vi "PARSER.vi"() -> ()   [LabVIEW 2010]
panel:
  out "HTTP Header":string
  out "Path":string
  out "Config":cluster{"OpenFP":bool, "UseAuthentication":bool}
  out "errors":errorcluster
  out "ControlIndicator":T1(array[cluster])
  out "vi reference":refnum<vi>
  out "SesionID":i32
  out "JIL-XMLversion":string="Version 0.1"
  out "STATE":T2(ring)
  out "Compatible utf8?":bool
  out "Commands recieved":i32
  out "IMPUT":string
  out "OUTPUT":string
  out "Error TCP":errorcluster
  in  "CloneRef":refnum<vi>
  in  "connection ID":refnum<k5>
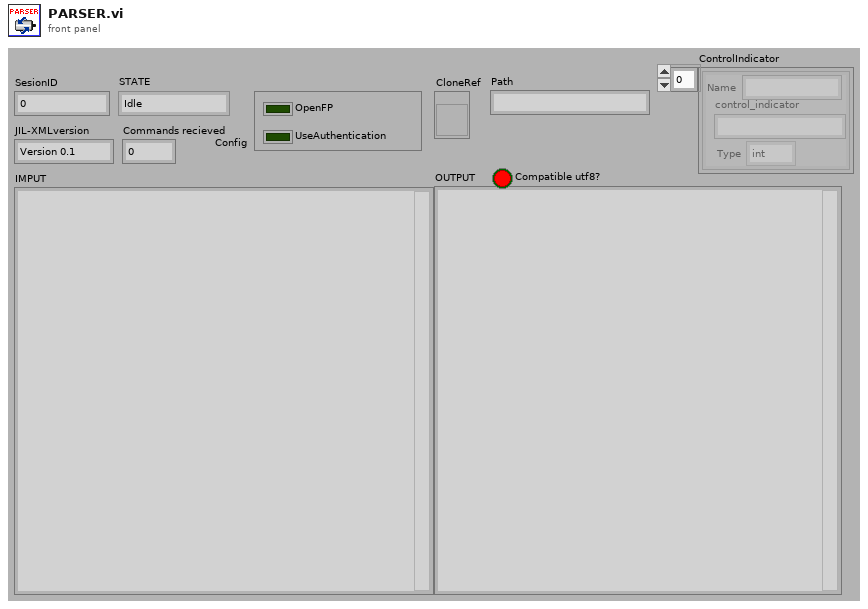
[diagram p1: front panel]
types:
  T1 = cluster{"Name":string, "control_indicator":string, "Type":enum16{"int", "boolean", "string", "double", "dateTime", "base64", "struct", "array"}}[]
  T2 = enum16{"Idle", "Connected", "Authenticated", "Opened", "Running", "Exit"}
  T3 = enum16{"Standard", "Buffered", "CRLF", "Immediate"}
  T4 = enum16{"Connect", "Authenticate", "OpenVI", "RunVI", "SyncVI", "StopVI", "CloseVI", "Disconnect"}
  T5 = enum16{"int", "boolean", "string", "double", "dateTime", "base64", "struct", "array"}
  T6 = enum16{"Update", "registry", "Init", "clean", "Close"}
  T7 = enum16{"int", "boolean", "string", "double", "dateTime", "base64", "struct", "array"}[]
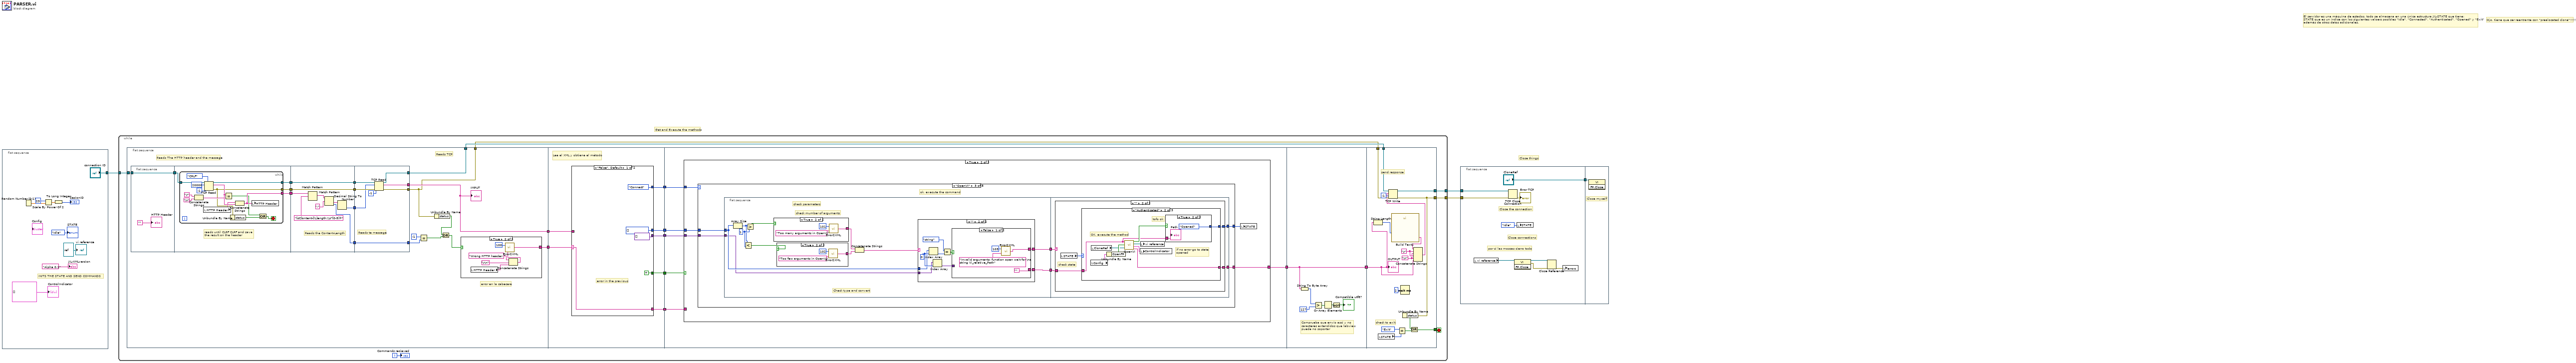
[diagram p0: block diagram]
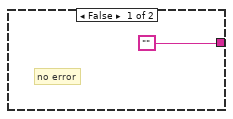
[diagram p2: hidden frame]
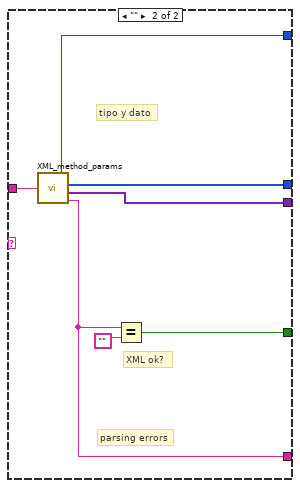
[diagram p3: hidden frame]
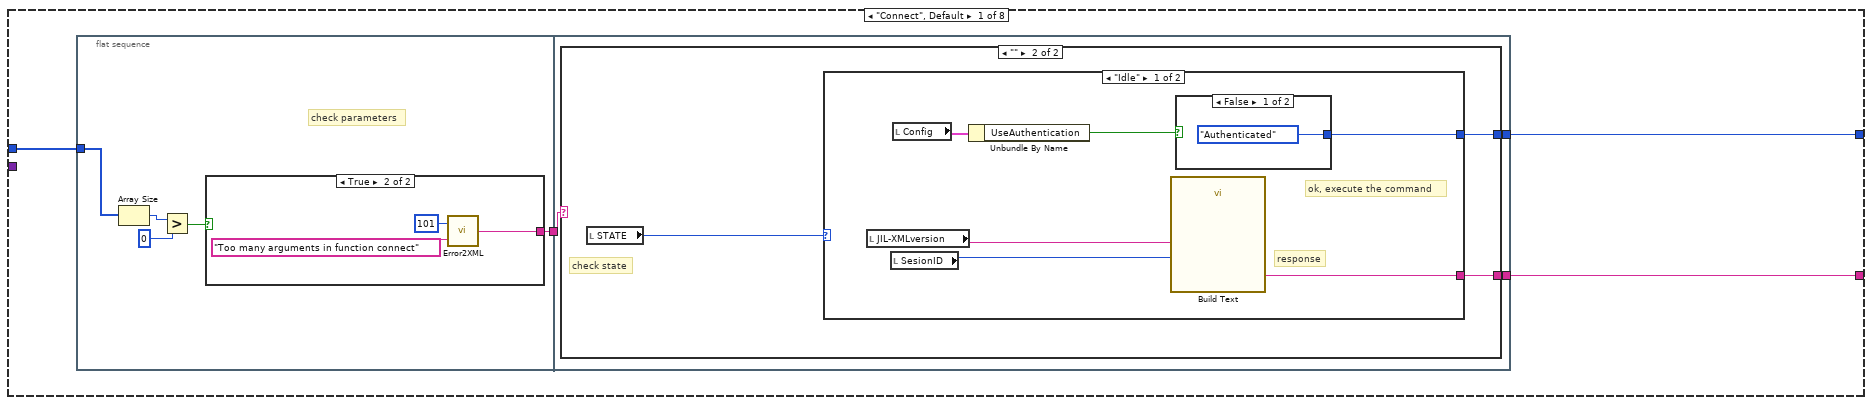
[diagram p5: hidden frame]
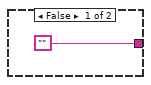
[diagram p6: hidden frame]
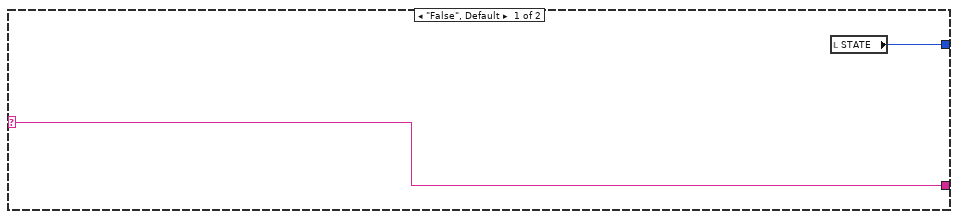
[diagram p7: hidden frame]
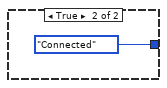
[diagram p8: hidden frame]
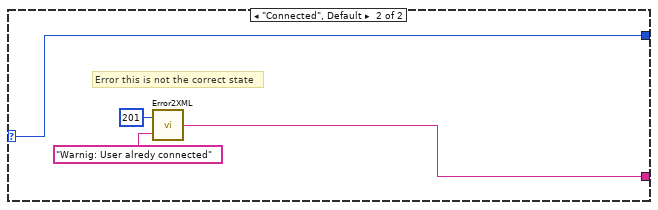
[diagram p9: hidden frame]
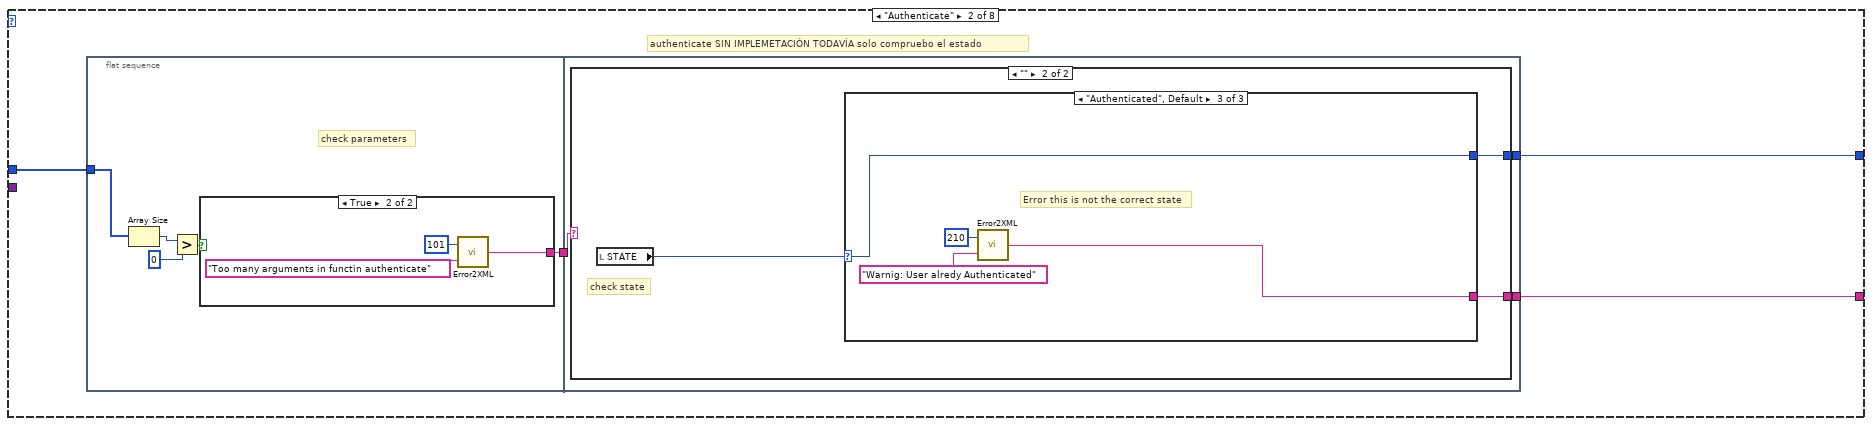
[diagram p10: hidden frame]
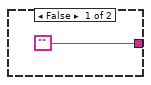
[diagram p11: hidden frame]
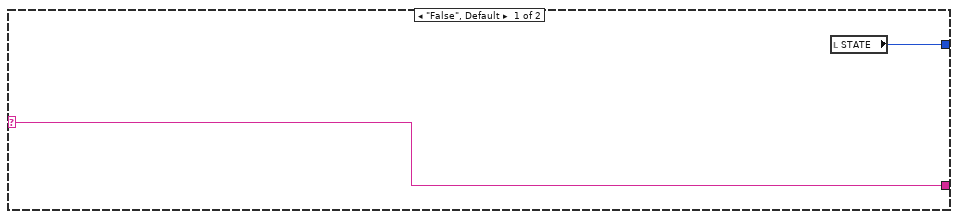
[diagram p12: hidden frame]
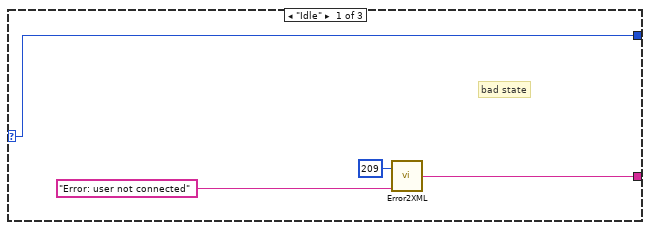
[diagram p13: hidden frame]
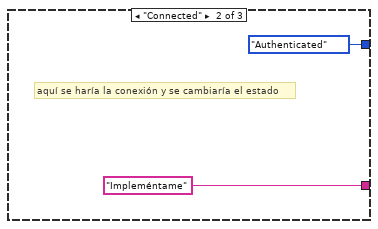
[diagram p14: hidden frame]
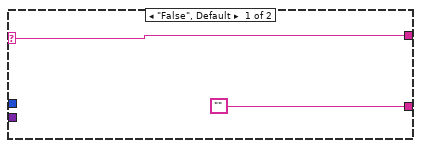
[diagram p15: hidden frame]
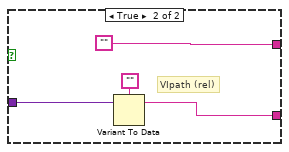
[diagram p16: hidden frame]
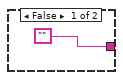
[diagram p17: hidden frame]
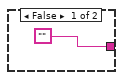
[diagram p18: hidden frame]
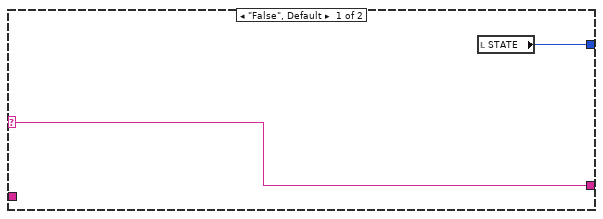
[diagram p19: hidden frame]
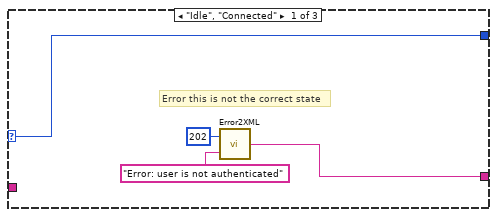
[diagram p20: hidden frame]
diagram:
  # "Close things"
  # "Get and Execute the methods"
  # "El servidor es una máquina de estados, todo se almacena en una única estructura JIL-STATE que tiene:\nSTATE que es un índice con los siguientes valoers posibles \"Idle\", \"Connected\", \"Authenticated\", \"Opened\" y \"Exit\"\nademás de otros datos adicionales."
  # "Ojo, tiene que ser reentrante con \"prealocated clone\"!!!!!!"
  n1 = flat-sequence {
    tunnel: ["connection ID"] -> w1
    frame #0 {
      # "INITS THE STATE AND SEND COMMANDS"
      n2 = Random Number (0-1)() -> (number: 0 to 1=w9:dbl)
      n3 = Scale By Power Of 2(n=23, x=w9) -> (x*2^n=w10:dbl)
      n4 = To Long Integer(number=w10) -> (32bit integer=→"SesionID":i32)
      "STATE" <- T2."Idle" ("STATE")
      "JIL-XMLversion" <- "Alpha 0.1" ("JIL-XMLversion")
      "vi reference" <- refnum<vi> refnum ("vi reference")
      "ControlIndicator" <- T1 [] ("ControlIndicator")
    }
  }
  n5 = while {
    tunnel: [w29] -> w3
    tunnel: [w26] -> w2
    tunnel: w1 -> [w15]
    i -> [w24]
    stop <- w27 stop-if-true
    n6 = flat-sequence {
      tunnel: [w39] -> w28
      tunnel: [w37] -> w25
      tunnel: [w38] -> w21
      tunnel: w15 -> [w47]
      tunnel: [w30] -> w14
      tunnel: [w95] -> w23
      tunnel: [w94] -> w22
      tunnel: w21 -> [w99]
      tunnel: [w98] -> w20
      tunnel: [w97] -> w18
      tunnel: [w96] -> w17
      tunnel: w14 -> [w93]
      tunnel: w23 -> [w117]
      tunnel: [w115] -> w19
      tunnel: w22 -> [w116]
      tunnel: w20 -> [w114]
      tunnel: w18 -> [w113]
      tunnel: w17 -> [w112]
      tunnel: w19 -> [w478]
      tunnel: [w478] -> w16
      tunnel: [w491] -> w29
      tunnel: w28 -> [w492]
      tunnel: [w495] -> w27
      tunnel: [w494] -> w26
      tunnel: w25 -> [w498]
      tunnel: w16 -> [w483]
      frame #0 {
        # "error en la cabecera"
        # "Reads The HTTP header and the message"
        # "Reads TCP"
        n7 = flat-sequence {
          tunnel: w47 -> [w55]
          tunnel: [w55] -> w46
          tunnel: w46 -> [w60]
          tunnel: [w59] -> w45
          tunnel: [w58] -> w42
          tunnel: [w57] -> w40
          tunnel: w45 -> [w84]
          tunnel: [w79] -> w44
          tunnel: [w78] -> w43
          tunnel: w42 -> [w78]
          tunnel: [w77] -> w41
          tunnel: w40 -> [w77]
          tunnel: [w76] -> w36
          tunnel: w44 -> [w89]
          tunnel: w43 -> [w90]
          tunnel: w41 -> [w91]
          tunnel: [w88] -> w39
          tunnel: [w87] -> w37
          tunnel: [w86] -> w38
          tunnel: [w85] -> w35
          tunnel: w36 -> [w85]
          frame #0 {
            "HTTP Header" <- ""
          }
          frame #1 {
            # "reads until CLRF CLRF and save \nthe result on the header"
            n8 = while {
              tunnel: w60 -> [w74]
              tunnel: [w66] -> w59
              tunnel: [w64] -> w58
              tunnel: [w65] -> w57
              stop <- w61 stop-if-true
              n9 = Concatenate Strings("\r", "\n") -> (w69:string)
              n10 = local read "HTTP Header"() -> (w70:string)
              n11 = TCP Read(connection ID=w74, bytes to read=20000, 7:T3."CRLF" ("mode (standard)"), 9:-1 ("timeout ms (25000)")) -> (connection ID out=w65:refnum<k5>, data out=w71:string, error out=w64:errorcluster)  [unwired: 1 in]
              n12 = Equal?(x=w71, y=w69) -> (x = y?=w63:bool)
              n13 = Unbundle By Name(w64) -> ("status"=w62:bool)
              n14 = Concatenate Strings(w70, w71) -> (w66:string)
              n15 = local write "HTTP Header"(w66) -> ()
              n16 = Or(x=w63, y=w62) -> (x .or. y?=w61:bool)
            }
          }
          frame #2 {
            # "Reads the Content-Length"
            n17 = Match Pattern(string=w84, regular expression="[cC]ontent-[lL]ength:\\s*[0-9]+") -> (match substring=w82:string)  [unwired: 1 in, 3 out]
            n18 = Match Pattern(string=w82, regular expression=":") -> (after substring=w80:string, offset past match=w76:i32)  [unwired: 1 in, 2 out]
            n19 = Decimal String To Number(string=w80) -> (number=w79:i32)  [unwired: 2 in, 1 out]
          }
          frame #3 {
            # "Reads te message"
            n20 = TCP Read(connection ID=w91, bytes to read=w89, error in (no error)=w90, 9:-1 ("timeout ms (25000)")) -> (connection ID out=w88:refnum<k5>, data out=w86:string, error out=w87:errorcluster)  [unwired: 1 in]
          }
        }
        n21 = Equal?(x=-1, y=w35) -> (x = y?=w33:bool)
        n22 = Unbundle By Name(w37) -> ("status"=w32:bool)
        n23 = Or(x=w32, y=w33) -> (x .or. y?=w31:bool)
        n24 = case shown="True" w31 {
          tunnel: ["" w53] -> w30
          frame False {
            # "no error"
          }
          frame True {
            n25 = local read "HTTP Header"() -> (w50:string)
            n26 = Concatenate Strings("Wrong HTTP header: ", "\r\n", w50) -> (w49:string)
            n27 = call "Error2XML.vi"("FailDescriptor"=w49, "FailID"=100) -> ("ErrorXML"=w53:string)
          }
        }
        "IMPUT" <- w38
      }
      frame #1 {
        # "Lee el XML y obtiene el método"
        n28 = case shown="\"False\", Default" w93 {
          selector: w93 -> [w104 _]
          tunnel: w99 -> [_ w111]
          tunnel: [TRUE w109] -> w98
          tunnel: [variant[] [] ("Values") w108] -> w97
          tunnel: [w102 w107] -> w96
          tunnel: [T4."Connect" ("Method") w106] -> w95
          tunnel: [w104 w105] -> w94
          frame "False", Default {
            w102 = T7 [] items=["int", "boolean", "string", "double", "dateTime", "base64", "struct", "array"] ("Types")
            # "error in the previous"
          }
          frame "" {
            # "parsing errors"
            # "tipo y dato"
            # "XML ok?"
            n29 = call "XML_method_params.vi"("XML-message"=w111) -> ("ParsingErrors"=w105:string, "Values"=w108:variant[], "Types"=w107:T7, "Method"=w106:T4)
            n30 = Equal?(x=w105, y="") -> (x = y?=w109:bool)
          }
        }
      }
      frame #2 {
        n31 = case shown="True" w114 {
          tunnel: w117 -> [_ w123]
          tunnel: w116 -> [w118 _]
          tunnel: [w118 w122] -> w115
          tunnel: w113 -> [_ w120]
          tunnel: w112 -> [_ w121]
          frame False {
            # "Returns the Parsing errors. Do not execute any method"
          }
          frame True {
            n32 = case shown="\"OpenVI\"" w123 {
              tunnel: [w125 w159 w192 w262 w313 w339 w388 w415] -> w122
              tunnel: w121 -> [w127 w158 w190 w264 w312 w341 w390 w418]
              tunnel: w120 -> [_ _ w189 _ _ _ _ w417]
              tunnel: [w124 w157 w191 w263 w311 w340 w389 w416] -> w119
              frame "Connect", Default {
                n33 = flat-sequence {
                  tunnel: w127 -> [w129]
                  tunnel: [w128] -> w126
                  tunnel: w126 -> [w139]
                  tunnel: [w138] -> w125
                  tunnel: [w137] -> w124
                  frame #0 {
                    # "check parameters"
                    n34 = Array Size(array=w129) -> (size(s)=w132:i32)
                    n35 = Greater?(x=w132, y=0) -> (0:w130:bool)
                    n36 = case shown="True" w130 {
                      tunnel: ["" w134] -> w128
                      frame False {
                      }
                      frame True {
                        n37 = call "Error2XML.vi"("FailDescriptor"="Too many arguments in function connect", "FailID"=101) -> ("ErrorXML"=w134:string)
                      }
                    }
                  }
                  frame #1 {
                    n38 = case shown="\"\"" w139 {
                      selector: w139 -> [w141 _]
                      tunnel: [w141 w144] -> w138
                      tunnel: [w140 w142] -> w137
                      frame "False", Default {
                        n39 = local read "STATE"() -> (w140:T2)
                      }
                      frame "" {
                        # "check state"
                        n40 = local read "STATE"() -> (w143:T2)
                        n41 = case shown="\"Idle\"" w143 {
                          selector: w143 -> [_ w153]
                          tunnel: [w150 w154] -> w144
                          tunnel: [w147 w153] -> w142
                          frame "Idle" {
                            # "ok, execute the command"
                            # "response"
                            n42 = local read "JIL-XMLversion"() -> (w148:string)
                            n43 = local read "SesionID"() -> (w149:i32)
                            n44 = local read "Config"() -> (w146:cluster{"OpenFP":bool, "UseAuthentication":bool})
                            n45 = Unbundle By Name(w146) -> ("UseAuthentication"=w145:bool)
                            n46 = call "Build Text"("JIL-XMLversion"=w148, "SessionID"=w149) -> ("Result"=w150:string)  [unwired: 12 in, 1 out]
                            n47 = case shown="False" w145 {
                              tunnel: [T2."Authenticated" ("STATE") T2."Connected" ("STATE")] -> w147
                              frame False {
                              }
                              frame True {
                              }
                            }
                          }
                          frame "Connected", Default {
                            # "Error this is not the correct state"
                            n48 = call "Error2XML.vi"("FailDescriptor"="Warnig: User alredy connected" ("FileDescriptor"), "FailID"=201) -> ("ErrorXML"=w154:string)
                          }
                        }
                      }
                    }
                  }
                }
              }
              frame "Authenticate" {
                # "authenticate SIN IMPLEMETACIÓN TODAVÍA solo compruebo el estado"
                n49 = flat-sequence {
                  tunnel: w158 -> [w162]
                  tunnel: [w161] -> w160
                  tunnel: w160 -> [w172]
                  tunnel: [w171] -> w159
                  tunnel: [w170] -> w157
                  frame #0 {
                    # "check parameters"
                    n50 = Array Size(array=w162) -> (size(s)=w165:i32)
                    n51 = Greater?(x=w165, y=0) -> (0:w163:bool)
                    n52 = case shown="True" w163 {
                      tunnel: ["" w167] -> w161
                      frame False {
                      }
                      frame True {
                        n53 = call "Error2XML.vi"("FailDescriptor"="Too many arguments in functin authenticate", "FailID"=101) -> ("ErrorXML"=w167:string)
                      }
                    }
                  }
                  frame #1 {
                    n54 = case shown="\"\"" w172 {
                      selector: w172 -> [w174 _]
                      tunnel: [w174 w177] -> w171
                      tunnel: [w173 w175] -> w170
                      frame "False", Default {
                        n55 = local read "STATE"() -> (w173:T2)
                      }
                      frame "" {
                        # "check state"
                        n56 = local read "STATE"() -> (w176:T2)
                        n57 = case shown="\"Authenticated\", Default" w176 {
                          selector: w176 -> [w178 _ w184]
                          tunnel: [w179 "Impleméntame" ("ErrorXML") w185] -> w177
                          tunnel: [w178 T2."Authenticated" ("STATE") w184] -> w175
                          frame "Idle" {
                            # "bad state"
                            n58 = call "Error2XML.vi"("FailDescriptor"="Error: user not connected", "FailID"=209) -> ("ErrorXML"=w179:string)
                          }
                          frame "Connected" {
                            # "aquí se haría la conexión y se cambiaría el estado"
                          }
                          frame "Authenticated", Default {
                            # "Error this is not the correct state"
                            n59 = call "Error2XML.vi"("FailDescriptor"="Warnig: User alredy Authenticated" ("FileDescriptor"), "FailID"=210) -> ("ErrorXML"=w185:string)
                          }
                        }
                      }
                    }
                  }
                }
              }
              frame "OpenVI" {
                # "ok, execute the command"
                n60 = flat-sequence {
                  tunnel: w190 -> [w195]
                  tunnel: [w198] -> w193
                  tunnel: w189 -> [w194]
                  tunnel: [w197] -> w188
                  tunnel: w193 -> [w235]
                  tunnel: [w234] -> w192
                  tunnel: [w233] -> w191
                  tunnel: w188 -> [w232]
                  frame #0 {
                    w202 = 1 ("y")
                    # "Check type and convert"
                    # "check mumber of arguments"
                    # "check parameters"
                    n61 = Array Size(array=w195) -> (size(s)=w201:i32)
                    n62 = Less?(x=w201, y=w202) -> (x < y?=w203:bool)
                    n63 = Greater?(x=w201, y=w202) -> (0:w204:bool)
                    n64 = case shown="True" w204 {
                      tunnel: ["" w229] -> w200
                      frame False {
                      }
                      frame True {
                        n65 = call "Error2XML.vi"("FailDescriptor"="Too many arguments in OpenVI", "FailID"=101) -> ("ErrorXML"=w229:string)
                      }
                    }
                    n66 = case shown="True" w203 {
                      tunnel: ["" w225] -> w199
                      frame False {
                      }
                      frame True {
                        n67 = call "Error2XML.vi"("FailDescriptor"="Too few arguments in OpenVI", "FailID"=102) -> ("ErrorXML"=w225:string)
                      }
                    }
                    n68 = Concatenate Strings(w200, w199) -> (w196:string)
                    n69 = case shown="\"\"" w196 {
                      selector: w196 -> [w206 _]
                      tunnel: [w206 w214] -> w198
                      tunnel: ["" w215] -> w197
                      tunnel: w195 -> [_ w212]
                      tunnel: w194 -> [_ w211]
                      frame "False", Default {
                      }
                      frame "" {
                        w213 = 0 ("index")
                        n70 = Index Array(array=w212, index=w213) -> (element=w209:T5)
                        n71 = Index Array(array=w211, index=w213) -> (element=w208:variant)
                        n72 = Equal?(x=T5."string" ("y"), y=w209) -> (x = y?=w207:bool)
                        n73 = case shown="False" w207 {
                          tunnel: ["" w222] -> w215
                          tunnel: [w217 ""] -> w214
                          tunnel: w208 -> [_ w220]
                          frame False {
                            n74 = call "Error2XML.vi"("FailDescriptor"="Invalid arguments: function open wait for \na string Vi_relative_Path", "FailID"=103) -> ("ErrorXML"=w217:string)
                          }
                          frame True {
                            # "VIpath (rel)"
                            n75 = Variant To Data(Variant=w220, type="") -> (data=w222:string)  [unwired: 1 in, 1 out]
                          }
                        }
                      }
                    }
                  }
                  frame #1 {
                    n76 = case shown="\"\"" w235 {
                      selector: w235 -> [w237 _]
                      tunnel: [w237 w241] -> w234
                      tunnel: [w236 w239] -> w233
                      tunnel: w232 -> [_ w238]
                      frame "False", Default {
                        n77 = local read "STATE"() -> (w236:T2)
                      }
                      frame "" {
                        # "check state"
                        n78 = local read "STATE"() -> (w240:T2)
                        n79 = case shown="\"Authenticated\"" w240 {
                          selector: w240 -> [w242 _ w261]
                          tunnel: [w243 w251 w258] -> w241
                          tunnel: [w242 w254 w261] -> w239
                          tunnel: w238 -> [_ w246 _]
                          frame "Idle", "Connected" {
                            # "Error this is not the correct state"
                            n80 = call "Error2XML.vi"("FailDescriptor"="Error: user is not authenticated" ("FileDescriptor"), "FailID"=202) -> ("ErrorXML"=w243:string)
                          }
                          frame "Authenticated" {
                            # "tofo ok"
                            # "if no error go to state\nopened"
                            # "OK, execute the method"
                            n81 = local read "Config"() -> (w250:cluster{"OpenFP":bool, "UseAuthentication":bool})
                            n82 = local read "CloneRef"() -> (w247:refnum<vi>)
                            n83 = Unbundle By Name(w250) -> ("OpenFP"=w249:bool)
                            n84 = call "OpenVI.vi"("CloneRef"=w247, "OpenFP"=w249, "Vi_relative_Path"=w246) -> ("ResponseXML"=w251:string, "ControlIndicator"=w252:T1, "vi reference"=w248:refnum<vi>, "OpenedOK?"=w253:bool)
                            n85 = local write "ControlIndicator"(w252) -> ()
                            n86 = local write "vi reference"(w248) -> ()
                            n87 = case shown="True" w253 {
                              tunnel: [T2."Authenticated" ("STATE") T2."Opened" ("STATE")] -> w254
                              tunnel: w246 -> [_ w256]
                              frame False {
                              }
                              frame True {
                                "Path" <- w256
                              }
                            }
                          }
                          frame "Opened", Default {
                            # "Error this is not the correct state"
                            n88 = call "Error2XML.vi"("FailDescriptor"="Error: There is a vi alredy opened." ("FileDescriptor"), "FailID"=203) -> ("ErrorXML"=w258:string)
                          }
                        }
                      }
                    }
                  }
                }
              }
              frame "RunVI" {
                # "IMPLEMENTA ALGO"
                n89 = flat-sequence {
                  tunnel: w264 -> [w267]
                  tunnel: [w266] -> w265
                  tunnel: w265 -> [w277]
                  tunnel: [w276] -> w262
                  tunnel: [w275] -> w263
                  frame #0 {
                    # "check parameters"
                    n90 = Array Size(array=w267) -> (size(s)=w270:i32)
                    n91 = Greater?(x=w270, y=0) -> (0:w268:bool)
                    n92 = case shown="True" w268 {
                      tunnel: ["" w272] -> w266
                      frame False {
                      }
                      frame True {
                        n93 = call "Error2XML.vi"("FailDescriptor"="Too many arguments in RunVI", "FailID"=101) -> ("ErrorXML"=w272:string)
                      }
                    }
                  }
                  frame #1 {
                    n94 = case shown="\"\"" w277 {
                      selector: w277 -> [w279 _]
                      tunnel: [w279 w282] -> w276
                      tunnel: [w278 w280] -> w275
                      frame "False", Default {
                        n95 = local read "STATE"() -> (w278:T2)
                      }
                      frame "" {
                        # "check state"
                        n96 = local read "STATE"() -> (w281:T2)
                        n97 = case shown="\"Opened\"" w281 {
                          selector: w281 -> [_ w303 w310]
                          tunnel: [w290 w304 w309] -> w282
                          tunnel: [w291 w303 w310] -> w280
                          frame "Opened" {
                            w289 = FALSE ("Wait Until Done")
                            n98 = local read "vi reference"() -> (w287:refnum<vi>)
                            n99 = property class="VI" props=["Front Panel.Open"](reference=w287) -> (reference out=w288:refnum<vi>, error out=w286:errorcluster)  [unwired: 1 in, 1 out]
                            n100 = invoke class="VI" method="Run VI"(reference=w288, error in=w286, "Wait until done"=w289, "Auto Dispose Ref"=w289) -> (reference out=w284:refnum<vi>, error out=w283:errorcluster)  [unwired: 1 in, 3 out]
                            n101 = Unbundle By Name(w283) -> ("status"=w285:bool)
                            n102 = case shown="False" w285 {
                              tunnel: [T2."Running" ("STATE") T2."Authenticated" ("STATE")] -> w291
                              tunnel: ["<?xml version=\"1.0\" encoding=\"UTF-8\"?>\n<methodResponse>\n\t<params>\n\t\t<param>\n\t\t\t<value><string>VI running</string></value>\n\t\t</param>\n\t</params>\n</methodResponse>\n" ("ErrorXML") w302] -> w290
                              tunnel: w284 -> [_ w299]
                              tunnel: w283 -> [_ w298]
                              frame False {
                                # "ok, command executed"
                              }
                              frame True {
                                # "weird fail, close the reference"
                                n103 = invoke class="VI" method="FP.Close"(reference=w299, error in=w298) -> (reference out=w297:refnum<vi>, error out=w296:errorcluster)  [unwired: 1 in, 1 out]
                                n104 = Close Reference(reference=w297, error in (no error)=w296) -> (error out=→"errors":errorcluster)
                                n105 = call "Error2XML.vi"("FailDescriptor"="Unexpected error: Vi cannot be run, Vi closed for safety reasons.", "FailID"=401) -> ("ErrorXML"=w302:string)
                              }
                            }
                          }
                          frame "Running" {
                            # "Error this is not the correct state"
                            n106 = call "Error2XML.vi"("FailDescriptor"="Error: Vi is running." ("FileDescriptor"), "FailID"=205) -> ("ErrorXML"=w304:string)
                          }
                          frame "Idle", Default {
                            n107 = call "Error2XML.vi"("FailDescriptor"="Error runing: Vi is not opened.", "FailID"=204) -> ("ErrorXML"=w309:string)
                          }
                        }
                      }
                    }
                  }
                }
              }
              frame "StopVI" {
                # "IMPLEMENTA ALGO"
                n108 = flat-sequence {
                  tunnel: w312 -> [w316]
                  tunnel: [w315] -> w314
                  tunnel: w314 -> [w326]
                  tunnel: [w325] -> w313
                  tunnel: [w324] -> w311
                  frame #0 {
                    # "check parameters"
                    n109 = Array Size(array=w316) -> (size(s)=w319:i32)
                    n110 = Greater?(x=w319, y=0) -> (0:w317:bool)
                    n111 = case shown="True" w317 {
                      tunnel: ["" w321] -> w315
                      frame False {
                      }
                      frame True {
                        n112 = call "Error2XML.vi"("FailDescriptor"="Too many arguments in StopVI", "FailID"=101) -> ("ErrorXML"=w321:string)
                      }
                    }
                  }
                  frame #1 {
                    n113 = case shown="\"\"" w326 {
                      selector: w326 -> [w328 _]
                      tunnel: [w328 w331] -> w325
                      tunnel: [w327 w329] -> w324
                      frame "False", Default {
                        n114 = local read "STATE"() -> (w327:T2)
                      }
                      frame "" {
                        # "check state"
                        n115 = local read "STATE"() -> (w330:T2)
                        n116 = case shown="\"Running\"" w330 {
                          selector: w330 -> [_ w338]
                          tunnel: [w334 w337] -> w331
                          tunnel: [w333 w338] -> w329
                          frame "Running" {
                            # "ok, execute the command"
                            n117 = local read "vi reference"() -> (w332:refnum<vi>)
                            n118 = call "StopVI.vi"("vi reference in"=w332) -> ("responseXML"=w334:string, "STATE"=w333:T2)
                          }
                          frame "Idle", Default {
                            n119 = call "Error2XML.vi"("FailDescriptor"="Error stopping: Vi is not running.", "FailID"=206) -> ("ErrorXML"=w337:string)
                          }
                        }
                      }
                    }
                  }
                }
              }
              frame "CloseVI" {
                n120 = flat-sequence {
                  tunnel: w341 -> [w344]
                  tunnel: [w343] -> w342
                  tunnel: w342 -> [w354]
                  tunnel: [w353] -> w339
                  tunnel: [w352] -> w340
                  frame #0 {
                    # "check parameters"
                    n121 = Array Size(array=w344) -> (size(s)=w347:i32)
                    n122 = Greater?(x=w347, y=0) -> (0:w345:bool)
                    n123 = case shown="True" w345 {
                      tunnel: ["" w349] -> w343
                      frame False {
                      }
                      frame True {
                        n124 = call "Error2XML.vi"("FailDescriptor"="Too many arguments in CloseVI", "FailID"=101) -> ("ErrorXML"=w349:string)
                      }
                    }
                  }
                  frame #1 {
                    n125 = case shown="\"\"" w354 {
                      selector: w354 -> [w356 _]
                      tunnel: [w356 w359] -> w353
                      tunnel: [w355 w357] -> w352
                      frame "False", Default {
                        n126 = local read "STATE"() -> (w355:T2)
                      }
                      frame "" {
                        # "check state"
                        n127 = local read "STATE"() -> (w358:T2)
                        n128 = case shown="\"Opened\"" w358 {
                          selector: w358 -> [_ w380 w384]
                          tunnel: [w365 w381 w385] -> w359
                          tunnel: [T2."Authenticated" ("STATE") w380 w384] -> w357
                          frame "Opened" {
                            # "update registry"
                            # "ok, execute the command"
                            # "response"
                            n129 = local read "vi reference"() -> (w364:refnum<vi>)
                            n130 = local read "CloneRef"() -> (w363:refnum<vi>)
                            n131 = property class="VI" props=["Front Panel.Open"](reference=w364) -> (reference out=w369:refnum<vi>, error out=w368:errorcluster)  [unwired: 1 in, 1 out]
                            n132 = call "Registry.vi"("OpenedVI"=cluster{"ViReference":refnum<vi>, "Path":string} {"ViReference"=refnum, "Path"=""}, "ParserReferecne"=w363, "Command"=T6."Update") -> ()  [unwired: 1 in, 3 out]
                            n133 = invoke class="VI" method="FP.Close"(reference=w369, error in=w368) -> (reference out=w367:refnum<vi>, error out=w366:errorcluster)  [unwired: 1 in, 1 out]
                            n134 = local write "Path"("") -> ()
                            n135 = case shown="Error" w366 {
                              selector: w366 -> [_ w374]
                              tunnel: [T2."Authenticated" ("STATE") T2."Authenticated" ("STATE")] -> _
                              tunnel: ["<?xml version=\"1.0\" encoding=\"UTF-8\"?>\n<methodResponse>\n\t<params>\n\t\t<param>\n\t\t\t<value><string>Vi closed sucesfully</string></value>\n\t\t</param>\n\t</params>\n</methodResponse>" ("ErrorXML") w379] -> w365
                              tunnel: w367 -> [_ w375]
                              frame No Error {
                                # "todo ok"
                                # "ok, command executed"
                              }
                              frame Error {
                                # "weird fail, close the reference"
                                n136 = Close Reference(reference=w375, error in (no error)=w374) -> (error out=w373:errorcluster)
                                n137 = call "Error2XML.vi"("FailDescriptor"="Unexpected error during close.", "FailID"=601) -> ("ErrorXML"=w379:string)
                                n138 = local write "errors"(w373) -> ()
                              }
                            }
                          }
                          frame "Running" {
                            # "Error this is not the correct state"
                            n139 = call "Error2XML.vi"("FailDescriptor"="Error: Vi is running stop it firs" ("FileDescriptor"), "FailID"=207) -> ("ErrorXML"=w381:string)
                          }
                          frame "Connected", Default {
                            # "Error this is not the correct state"
                            n140 = call "Error2XML.vi"("FailDescriptor"="Error closing: Vi is not opened." ("FileDescriptor"), "FailID"=208) -> ("ErrorXML"=w385:string)
                          }
                        }
                      }
                    }
                  }
                }
              }
              frame "Disconnect" {
                n141 = flat-sequence {
                  tunnel: w390 -> [w393]
                  tunnel: [w392] -> w391
                  tunnel: w391 -> [w403]
                  tunnel: [w402] -> w388
                  tunnel: [w401] -> w389
                  frame #0 {
                    # "check parameters"
                    n142 = Array Size(array=w393) -> (size(s)=w396:i32)
                    n143 = Greater?(x=w396, y=0) -> (0:w394:bool)
                    n144 = case shown="True" w394 {
                      tunnel: ["" w398] -> w392
                      frame False {
                      }
                      frame True {
                        n145 = call "Error2XML.vi"("FailDescriptor"="Too many arguments in disconnect", "FailID"=101) -> ("ErrorXML"=w398:string)
                      }
                    }
                  }
                  frame #1 {
                    n146 = case shown="\"\"" w403 {
                      selector: w403 -> [w405 _]
                      tunnel: [w405 w408] -> w402
                      tunnel: [w404 w406] -> w401
                      frame "False", Default {
                        n147 = local read "STATE"() -> (w404:T2)
                      }
                      frame "" {
                        # "check state"
                        n148 = local read "STATE"() -> (w407:T2)
                        n149 = case shown="\"Connected\", Default" w407 {
                          selector: w407 -> [_ w411]
                          tunnel: ["<?xml version=\"1.0\" encoding=\"UTF-8\"?>\n<methodResponse>\n\t<params>\n\t\t<param>\n\t\t\t<value><string>See you soon</string></value>\n\t\t</param>\n\t</params>\n</methodResponse>\n" ("ErrorXML") w412] -> w408
                          tunnel: [T2."Exit" ("STATE") w411] -> w406
                          frame "Connected", Default {
                            # "ok, execute the command"
                          }
                          frame "Opened", "Running" {
                            # "Error this is not the correct state"
                            n150 = call "Error2XML.vi"("FailDescriptor"="Error: There is a Vi opened close it before disconnecting." ("FileDescriptor"), "FailID"=209) -> ("ErrorXML"=w412:string)
                          }
                        }
                      }
                    }
                  }
                }
              }
              frame "SyncVI" {
                n151 = flat-sequence {
                  tunnel: w418 -> [w422]
                  tunnel: [w425] -> w420
                  tunnel: w417 -> [w421]
                  tunnel: [w424] -> w419
                  tunnel: w420 -> [w460]
                  tunnel: [w459] -> w415
                  tunnel: [w458] -> w416
                  tunnel: w419 -> [w457]
                  frame #0 {
                    w429 = 1 ("y")
                    # "Check type and convert"
                    # "check mumber of arguments"
                    # "check parameters"
                    n152 = Array Size(array=w422) -> (size(s)=w428:i32)
                    n153 = Less?(x=w428, y=w429) -> (x < y?=w430:bool)
                    n154 = Greater?(x=w428, y=w429) -> (0:w431:bool)
                    n155 = case shown="True" w431 {
                      tunnel: ["" w454] -> w427
                      frame False {
                      }
                      frame True {
                        n156 = call "Error2XML.vi"("FailDescriptor"="Too many arguments in SyncVI", "FailID"=101) -> ("ErrorXML"=w454:string)
                      }
                    }
                    n157 = case shown="True" w430 {
                      tunnel: ["" w450] -> w426
                      frame False {
                      }
                      frame True {
                        n158 = call "Error2XML.vi"("FailDescriptor"="Too few arguments in SyncVI", "FailID"=102) -> ("ErrorXML"=w450:string)
                      }
                    }
                    n159 = Concatenate Strings(w427, w426) -> (w423:string)
                    n160 = case shown="\"\"" w423 {
                      selector: w423 -> [w433 _]
                      tunnel: [w433 w441] -> w425
                      tunnel: ["" w442] -> w424
                      tunnel: w422 -> [_ w439]
                      tunnel: w421 -> [_ w438]
                      frame "False", Default {
                      }
                      frame "" {
                        w440 = 0 ("index")
                        n161 = Index Array(array=w439, index=w440) -> (element=w436:T5)
                        n162 = Index Array(array=w438, index=w440) -> (element=w435:variant)
                        n163 = Equal?(x=T5."array" ("y"), y=w436) -> (x = y?=w434:bool)
                        n164 = case shown="True" w434 {
                          tunnel: ["" w447] -> w442
                          tunnel: [w444 ""] -> w441
                          tunnel: w435 -> [_ w447]
                          frame False {
                            n165 = call "Error2XML.vi"("FailDescriptor"="Invalid arguments: function Sync wait for \na Array of clusters", "FailID"=103) -> ("ErrorXML"=w444:string)
                          }
                          frame True {
                          }
                        }
                      }
                    }
                  }
                  frame #1 {
                    n166 = case shown="\"\"" w460 {
                      selector: w460 -> [w462 _]
                      tunnel: [w462 w466] -> w459
                      tunnel: [w461 w464] -> w458
                      tunnel: w457 -> [_ w463]
                      frame "False", Default {
                        n167 = local read "STATE"() -> (w461:T2)
                      }
                      frame "" {
                        # "check state"
                        n168 = local read "STATE"() -> (w465:T2)
                        n169 = case shown="\"Opened\", \"Running\"" w465 {
                          selector: w465 -> [w467 w475]
                          tunnel: [w468 w472] -> w466
                          tunnel: [w467 w475] -> w464
                          tunnel: w463 -> [w471 _]
                          frame "Opened", "Running" {
                            # "OK, execute the method"
                            n170 = local read "vi reference"() -> (w470:refnum<vi>)
                            n171 = local read "ControlIndicator"() -> (w469:T1)
                            n172 = call "SyncVI.vi"("ControlIndicator"=w469, "vi reference"=w470, "ArrayOfComands"=w471) -> ("Response"=w468:string)  [unwired: 2 in]
                          }
                          frame "Idle", Default {
                            # "Error this is not the correct state"
                            n173 = call "Error2XML.vi"("FailDescriptor"="Error: Vi is not opened/running." ("FileDescriptor"), "FailID"=210) -> ("ErrorXML"=w472:string)
                          }
                        }
                      }
                    }
                  }
                }
              }
            }
            n174 = local write "STATE"(w119) -> ()
          }
        }
      }
      frame #3 {
        # "Comprueba que envío asci y no \ncaracteres extendidos que labview\npuede no soportar"
        n175 = String To Byte Array(string=w478) -> (unsigned byte array=w481:u8[])
        n176 = Greater?(x=w481, y=127) -> (0:w479:bool[])
        n177 = Or Array Elements(Boolean array=w479) -> (logical OR=w476:bool)
        n178 = Not(x=w476) -> (.not. x?=→"Compatible utf8?":bool)
      }
      frame #4 {
        w484 = "\n"
        w485 = "\r"
        # "check to exit"
        # "send response"
        n179 = String Length(string=w483) -> (length=w488:i32)
        n180 = local read "STATE"() -> (w490:T2)
        n181 = call "Build Text2"("longitud"=w488) -> ("Result"=w487:string)  [unwired: 13 in, 1 out]
        n182 = Equal?(x=T2."Exit", y=w490) -> (x = y?=w496:bool)
        n183 = Wait (ms)(milliseconds to wait=u32 2) -> ()  [unwired: 1 out]
        n184 = Concatenate Strings(w487, w485, w484, w485, w484, w483) -> (w486:string)
        n185 = TCP Write(connection ID=w492, data in=w486, error in (no error)=w498, 9:-1 ("timeout ms (25000)")) -> (connection ID out=w491:refnum<k5>, error out=w494:errorcluster)  [unwired: 1 out]
        n186 = Unbundle By Name(w494) -> ("status"=w493:bool)
        n187 = Or(x=w493, y=w496) -> (x .or. y?=w495:bool)
        "OUTPUT" <- w483
      }
    }
    "Commands recieved" <- w24
  }
  n188 = flat-sequence {
    tunnel: w3 -> [w507]
    tunnel: w2 -> [w505]
    tunnel: ["CloneRef"] -> w4
    tunnel: w4 -> [w508]
    frame #0 {
      # "por si las moscas cierro todo"
      # "Close connections"
      # "Close the connection"
      n189 = local read "vi reference"() -> (w499:refnum<vi>)
      n190 = TCP Close Connection(connection ID=w507, error in (no error)=w505) -> (error out=→"Error TCP":errorcluster)  [unwired: 1 in, 1 out]
      n191 = invoke class="VI" method="FP.Close"(reference=w499) -> (reference out=w502:refnum<vi>, error out=w501:errorcluster)  [unwired: 2 in, 1 out]
      n192 = local write "STATE"(T2."Idle" ("STATE")) -> ()
      n193 = Close Reference(reference=w502, error in (no error)=w501) -> (error out=w500:errorcluster)
      n194 = local write "errors"(w500) -> ()
    }
    frame #1 {
      # "Close myself"
      n195 = invoke class="VI" method="FP.Close"(reference=w508) -> ()  [unwired: 2 in, 3 out]
    }
  }
